vi "GetPowerN1911wHandle.vi"(2 "error in (no error)":errorcluster, 3 "connection ID":refnum<k5>) -> (0 "Error out":errorcluster, 1 "Power returned (dBm)":dbl format="%#.10f")   [LabVIEW 2009]
doc: "Reads the power from the N1911A power meter."
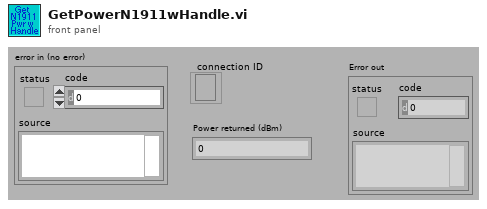
[diagram p1: front panel]
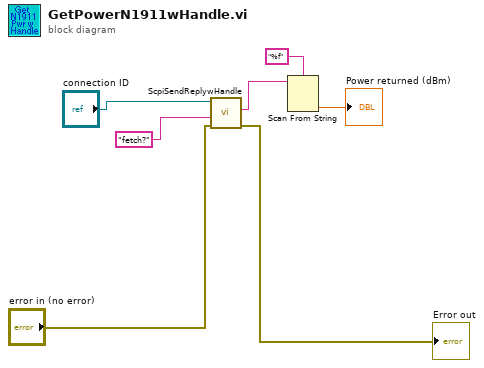
[diagram p0: block diagram]
diagram:
  n1 = call "ScpiSendReplywHandle.vi"("error in (no error)"="error in (no error)", "Command"="fetch?" ("format string"), "connection ID In"="connection ID") -> ("Error out"=→"Error out":errorcluster, "Reply"=w1:string)  [unwired: 5 in, 1 out]
  n2 = Scan From String(format string="%f", input string=w1) -> (output 1=→"Power returned (dBm)":dbl)  [unwired: 3 in, 3 out]
